vi "BH Druck PACE Series Process Filter.vi"() -> ()   [LabVIEW 2022 SP3]
uses:
  <vilib>/Utility/error.llb/DialogType.ctl
  BH Druck PACE Series.lvclass
panel:
  in  "Channel (0: Channel A)":u16(ring) items=["Channel A", "Channel B"]
  in  "Enable Filter (Off)":bool
  in  "Filter Band %FS":dbl=0.02 min=0.0 max=100.0 step=0.01
  in  "Filter Time (s)":dbl=2.0 min=0.0125 max=100.0 step=1.0
  in  "stop":bool
  out "Filter Time read (s)":dbl
  out "Filter Band Read":dbl
  out "Filter Status":bool
  in  "VISA resource name":refnum<visa-resource-name>
  # "(c)2010-2020 BH  Druck Ltd.  ALL RIGHTS RESERVED."
  # "Setup"
  # "Reading"
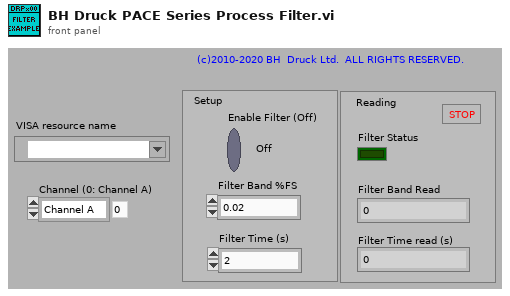
[diagram p1: front panel]
types:
  T1 = typedef "DialogType.ctl" = u16
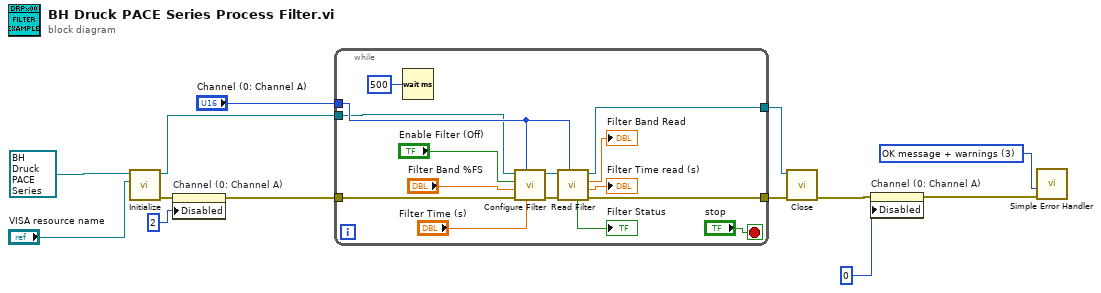
[diagram p0: block diagram]
diagram:
  w8 = T1 3 items=["no dialog", "OK message", "continue or stop message", "OK message + warnings", "continue/stop + warnings"] ("type of dialog (OK msg:1)")
  n1 = call-dynamic "Initialize.vi"("VISA resource name"="VISA resource name", "BH Druck PACE Series in"=refnum<class "BH Druck PACE Series.lvclass"> refnum) -> ("error out"=w3:errorcluster, "BH Druck PACE Series out"=w7:refnum<class "BH Druck PACE Series.lvclass">)  [unwired: 7 in]
  n2 = property on="Channel (0: Channel A)" class="Ring (strict)"(error in=w3, "Disabled"=u8 2) -> (error out=w6:errorcluster)  [unwired: 1 in, 1 out]
  n3 = while {
    tunnel: [w23] -> w13
    tunnel: [w24] -> w12
    tunnel: "Channel (0: Channel A)" -> [w25]
    tunnel: w7 -> [w22]
    tunnel: w6 -> [w21]
    stop <- "stop" stop-if-true
    n4 = Wait (ms)(milliseconds to wait=u32 500) -> ()  [unwired: 1 out]
    n5 = call-dynamic "Configure Filter.vi"("Filter Time (s) (2)"="Filter Time (s)", "Channel (0: Channel A)"=w25, "error in (no error)"=w21, "Filter Band %FS (0.02)"="Filter Band %FS", "Enable Filter (Off)"="Enable Filter (Off)", "BH Druck PACE Series in"=w22) -> ("error out"=w26:errorcluster, "BH Druck PACE Series out"=w27:refnum<class "BH Druck PACE Series.lvclass">)  [unwired: 4 in]
    n6 = call-dynamic "Read Filter.vi"("Channel (0: Channel A)"=w25, "error in (no error)"=w26, "BH Druck PACE Series in"=w27) -> ("error out"=w23:errorcluster, "Filter Time Read (s)"=→"Filter Time read (s)":dbl, "Filter Band Read"=→"Filter Band Read":dbl, "BH Druck PACE Series out"=w24:refnum<class "BH Druck PACE Series.lvclass">, "Filter Status"=→"Filter Status":bool)  [unwired: 4 in]
  }
  n7 = call "Close.vi"("error in (no error)"=w13, "BH Druck PACE Series in"=w12) -> ("error out"=w1:errorcluster)  [unwired: 8 in, 1 out]
  n8 = property on="Channel (0: Channel A)" class="Ring (strict)"(error in=w1, "Disabled"=u8 0) -> (error out=w9:errorcluster)  [unwired: 1 in, 1 out]
  n9 = call <vilib>:"Simple Error Handler.vi"("type of dialog (OK msg:1)"=w8, "error in (no error)"=w9) -> ()  [unwired: 3 in, 5 out]
